vi "NI PXI-4110 Programmable Power Supply RT Driver VI.vi"(6 "Device Clock":string, 9 "Device Inputs FIFO":refnum<k33>, 11 "Device Reference":T1 format="%.0x") -> ()   [LabVIEW 2018, in "NI PXI-4110 Programmable Power Supply Custom Device.lvlib"]
uses:
  NI PXI-4110 Programmable Power Supply Custom Device.lvlib
  <vilib>/NI Veristand/Custom Device API/Custom Device Item Ref.ctl
  <vilib>/NI Veristand/Custom Device API/Custom Device Channel Type.ctl
  <vilib>/Platform/TimedLoop/XDataNode/timing_clust.ctl
  <vilib>/Platform/TimedLoop/XDataNode/nitl_modes.ctl
  <vilib>/Platform/TimedLoop/XDataNode/wakeup.ctl
  4110_Channel #.ctl
  4110_Global.vi
  <vilib>/NI Veristand/Custom Device API/Get Item Property (Boolean).vi
  <vilib>/Platform/TimedLoop/XDataNode/XDataNode.xnode
  <vilib>/Platform/TimedLoop/XDataNode/XDNodeRunTimeDep.lvlib
  <vilib>/NI VeriStand/Custom Device API/Custom Device API.lvlib
  <vilib>/NI Veristand/Custom Device Tools/Custom Device Utility Library/Custom Device Utility Library.lvlib
panel:
  in  "Status Notifier":refnum<notifier>
  # "Custom Device Template\nv1.0"
  # "Use this template as a starting point for creating a custom device code module. The input controls shown here are specially named controls that the system will use to provide the device loop with data. The controls are not required for the device loop to run. For instance, if the device doesn't produce any output data, then you don't need the Device Outputs FIFO control. If you do use these controls, however, they need to have these exact names to be functional."
  # "The optional status notifier element is used to notify the RT engine of the last state of the custom device, and to indicate the device has completed execution. If this control is not used, a default No Error value is returned to the system when the device finishes execution.\n\nNote: This error state is not checked until the system shuts down. Use an output status channel to send more immediate status values to the system."
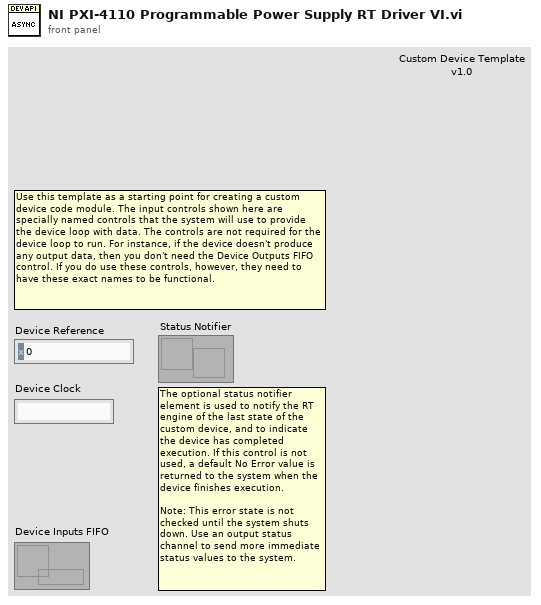
[diagram p1: front panel]
types:
  T1 = typedef "Custom Device API.lvlib/Custom Device Item Ref.ctl" = u64
  T2 = typedef "Custom Device API.lvlib/Custom Device Channel Type.ctl" = enum16{"Input", "Output"}
  T3 = typedef "Custom Device API.lvlib/Custom Device Timed Loop Priority.ctl" = enum32{"Low", "Medium", "High"}
  T4 = cluster{"instrument handle out":refnum<k15>, "Value":string, "Value":u16}[]
  T5 = typedef "XDNodeRunTimeDep.lvlib/timing_clust.ctl" = cluster{"Expected End [f-1]":u64, "Actual End [f-1]":u64, "Finished Late? [f-1]":bool, "Expected End [i-1]":u64, "Actual End [i-1]":u64, "Finished Late? [i-1]":bool, "Expected Start [i]":u64, "Actual Start [i]":u64, "Expected Start [f]":u64, "Actual Start [f]":u64, "Source Name":string, "Structure Name":string, "Period":i64, "Deadline":i64, "Offset":i64, "Start":i64, "Priority":i32, "Timeout":i32, "Mode":T6, "Wakeup Reason":T7, "Error":errorcluster, "Source Type":string, "Secondary Source Type":string, "Global End Time":u64, "Global Start Time":u64, "Frame Duration":u64, "Iteration Duration":u64, "Assigned CPU":i32, "I/O Scan Engine Mode":u32}
  T6 = typedef "XDNodeRunTimeDep.lvlib/nitl_modes.ctl" = enum32{"No Change", "Process missed periods, maintain original phase", "Discard missed periods, maintain original phase", "Process missed periods, ignore original phase", "Discard missed periods, ignore original phase"}
  T7 = typedef "XDNodeRunTimeDep.lvlib/wakeup.ctl" = enum32{"Normal", "Aborted", "Asynchronous wakeup", "Timing source error", "Timed loop error", "Timeout"}
  T8 = typedef "NI PXI-4110 Programmable Power Supply Custom Device.lvlib/4110_Channel #.ctl" = enum16{"0", "1", "2"}
  T9 = cluster{"V_min":dbl, "V_max":dbl, "I_min":dbl, "I_max":dbl}
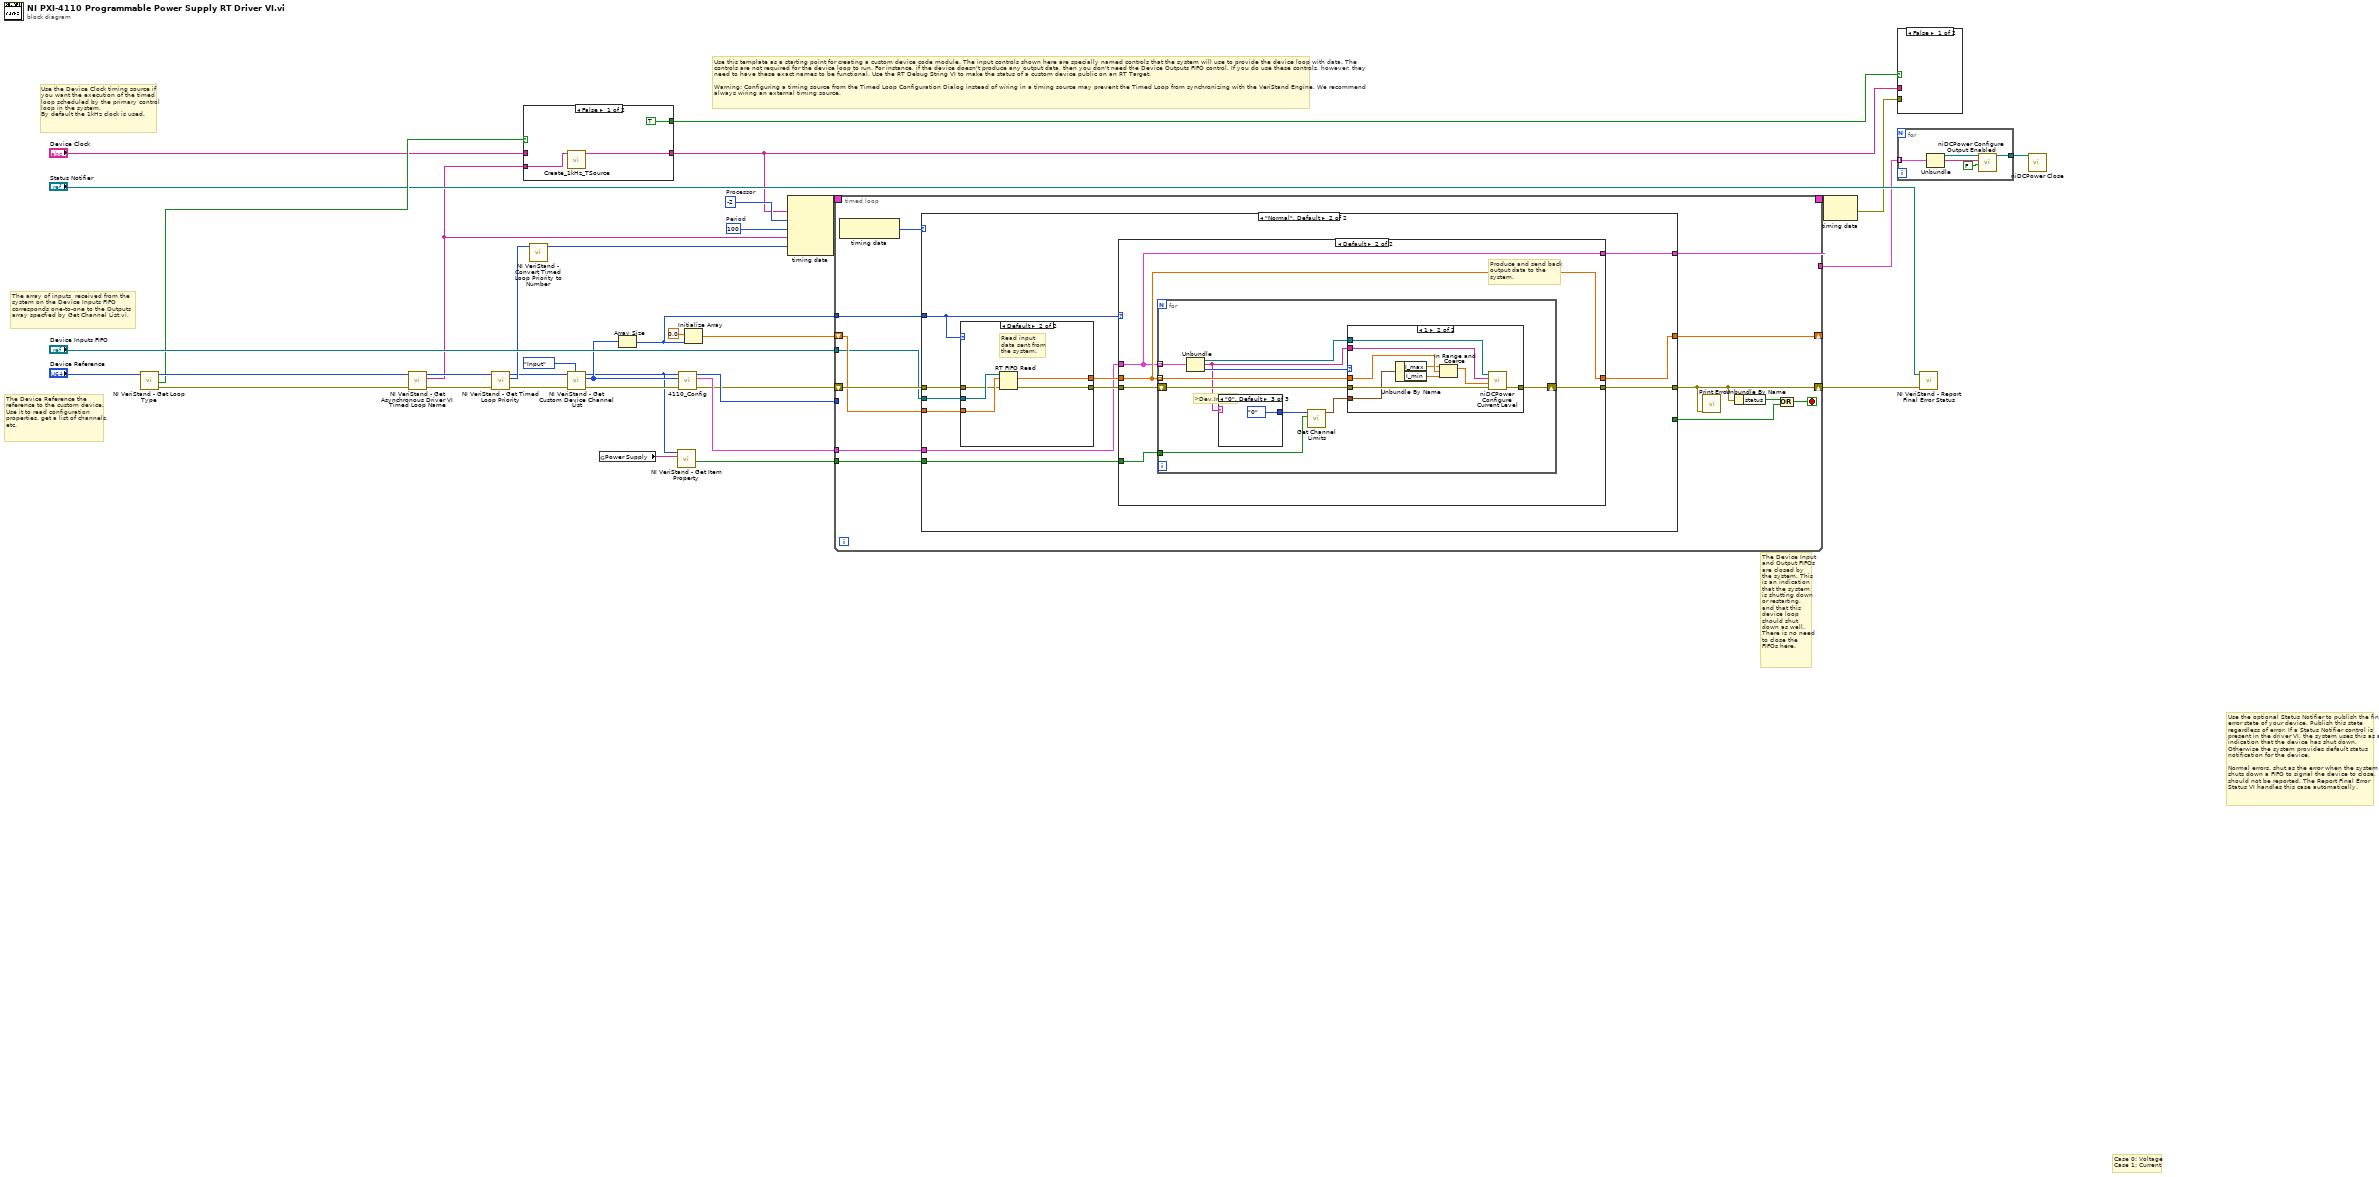
[diagram p0: block diagram]
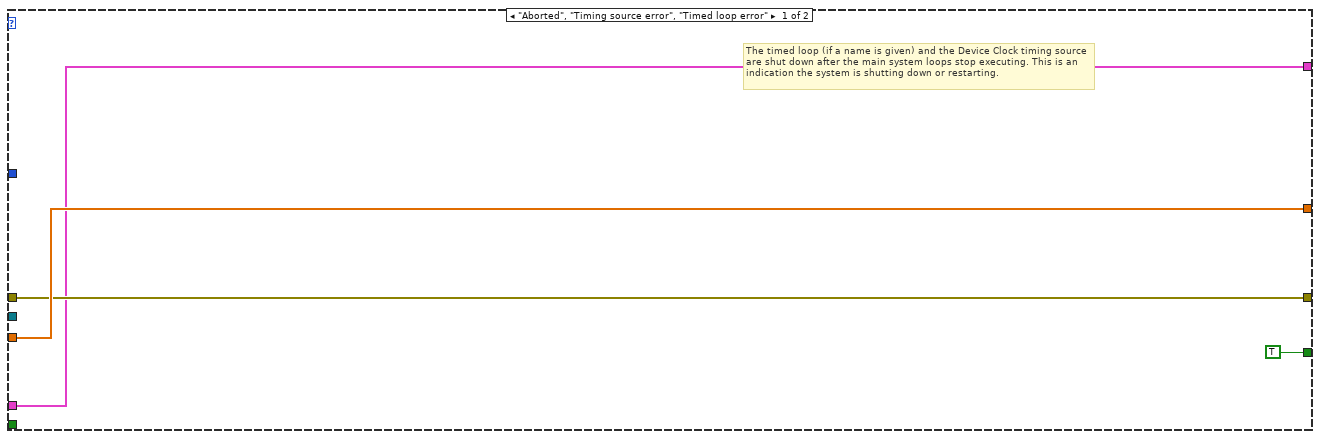
[diagram p2: hidden frame]
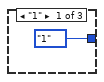
[diagram p4: hidden frame]
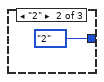
[diagram p5: hidden frame]
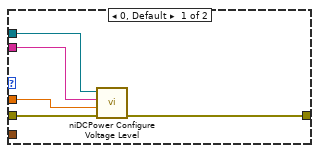
[diagram p6: hidden frame]
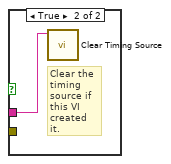
[diagram p9: hidden frame]
diagram:
  w26 = i64 100  # Period
  w27 = -2  # Processor
  # "Case 0: Voltage\nCase 1: Current"
  # "The array of inputs  received from the system on the Device Inputs FIFO corresponds one-to-one to the Outputs array specfied by Get Channel List.vi."
  # "Use the optional Status Notifier to publish the final error state of your device. Publish this state regardless of error. If a Status Notifier control is present in the driver VI, the system uses this as an indication that the device has shut down. Otherwise the system provides default status notification for the device.\n\nNormal errors, shut as the error when the system shuts down a FIFO to signal the device to close, should not be reported. The Report Final Error Status VI handles this case automatically."
  # "The Device Input and Output FIFOs are closed by the system. This is an indication that the system is shutting down or restarting, and that this device loop should shut down as well. There is no need to close the FIFOs here."
  # "The Device Reference the reference to the custom device. Use it to read configuration properties, get a list of channels, etc."
  # "Use the Device Clock timing source if you want the execution of the timed loop scheduled by the primary control loop in the system. \nBy default the 1kHz clock is used."
  # "Use this template as a starting point for creating a custom device code module. The input controls shown here are specially named controls that the system will use to provide the device loop with data. The controls are not required for the device loop to run. For instance, if the device doesn't produce any output data, then you don't need the Device Outputs FIFO control. If you do use these controls, however, they need to have these exact names to be functional. Use the RT Debug String VI to make the status of a custom device public on an RT Target.\n\nWarning: Configuring a timing source from the Timed Loop Configuration Dialog instead of wiring in a timing source may prevent the Timed Loop from synchronizing with the VeriStand Engine. We recommend always wiring an external timing source."
  n1 = call <vilib>:"NI VeriStand - Get Loop Type.vi"("Device Ref in"="Device Reference") -> ("error out"=w25:errorcluster, "Use Device Clock"=w22:bool, "Device Ref out"=w24:T1)  [unwired: 1 in, 7 out]
  n2 = call <vilib>:"NI VeriStand - Get Asynchronous Driver VI Timed Loop Name.vi"("error in (no error)"=w25, "Device Ref in"=w24) -> ("error out"=w30:errorcluster, "Device Timed Loop Name"=w16:string, "Device Ref out"=w36:T1)  [unwired: 7 out]
  n3 = call <vilib>:"NI VeriStand - Get Timed Loop Priority.vi"("error in (no error)"=w30, "Device Ref in"=w36) -> ("error out"=w4:errorcluster, "Priority"=w29:T3, "Device Ref out"=w15:T1)  [unwired: 7 out]
  n4 = case shown="False" w22 {
    tunnel: "Device Clock" -> [_ w40]
    tunnel: [w39 w40] -> w17
    tunnel: [TRUE _] -> w18
    tunnel: w16 -> [w37 _]
    frame False {
      n5 = call <vilib>:"Create_1kHz_TSource.vi"("name (in)"=w37) -> ("name (out)"=w39:string)  [unwired: 1 in, 9 out]
    }
    frame True {
    }
  }
  n6 = call <vilib>:"NI VeriStand - Convert Timed Loop Priority to Number.vi"("Priority"=w29) -> ("Numeric Priority"=w28:i32)  [unwired: 10 out]
  n7 = call <vilib>:"NI VeriStand - Get Custom Device Channel List.vi"("Channel Type"=Custom_Device_Channel_Type."Input", "error in (no error)"=w4, "Device Ref in"=w15) -> ("error out"=w12:errorcluster, "Specified Channel Ref List"=w13:T1[], "Device Ref out"=w2:T1)  [unwired: 6 out]
  n8 = global read "4110_Global.vi" "Power Supply"() -> (w3:string)
  n9 = Array Size(array=w13) -> (size(s)=w6:i32)
  n10 = call-poly <vilib>:"NI VeriStand - Get Item Property.vi"("Property Name"=w3, "Item Ref in"=w2) -> ("Value"=w1:bool)  [unwired: 6 in, 3 out]
  n11 = call "4110_Config.vi"("error in (no error)"=w12, "Specified Channel Ref List"=w13, "Device Ref out"=w2) -> ("error out"=w5:errorcluster, "Channel Info"=w11:T4, "Channel Ref List (out)"=w14:T1[])  [unwired: 6 in]
  n12 = Initialize Array(0.0 ("element"), w6) -> (w31:dbl[])
  n13 = node-c288(w17, w27, w26, w16, w28) -> (w34:T5)
  n14 = timed-loop {
    timing: w34 -> [_]
    timing-out: [_] -> w33
    shift-right: [w51] -> _
    shift-left: w31 -> [w52]
    shift-right: [w42] -> w9
    shift-left: w5 -> [w53]
    tunnel: "Device Inputs FIFO" -> [w49]
    tunnel: w6 -> [w45]
    tunnel: w14 -> [_]
    tunnel: w11 -> [w44]
    tunnel: [w43] -> w10
    tunnel: w1 -> [w41]
    stop <- w46 stop-if-true
    # ">Dev.Inputs>"
    n15 = node-c288() -> (w50:T7)  [unwired: 1 out]
    n16 = case shown="\"Normal\", Default" w50 {
      tunnel: w53 -> [w58 w65]
      tunnel: w52 -> [w59 w69]
      tunnel: [w58 w66] -> w42
      tunnel: [w59 w64] -> w51
      tunnel: w49 -> [_ w70]
      tunnel: [TRUE _] -> w47
      tunnel: w45 -> [_ w63]
      tunnel: w44 -> [w56 w62]
      tunnel: [w56 w61] -> w43
      tunnel: w41 -> [_ w60]
      frame "Aborted", "Timing source error", "Timed loop error" {
        # "The timed loop (if a name is given) and the Device Clock timing source are shut down after the main system loops stop executing. This is an indication the system is shutting down or restarting."
      }
      frame "Normal", Default {
        n17 = case shown="Default" w63 {
          tunnel: w70 -> [_ w112]
          tunnel: w69 -> [w107 w111]
          tunnel: [w107 w110] -> w68
          tunnel: [w106 w109] -> w67
          tunnel: w65 -> [w106 w108]
          frame 0 {
            # "No inputs to read\nfrom system. Inputs FIFO not created in this case, so don't write to it."
          }
          frame Default {
            # "Read input data sent from the system."
            n18 = RT FIFO Read(0:w112, 1:w111, 3:w108) -> (9:w110:dbl[], 11:w109:errorcluster)  [unwired: 4 out]
          }
        }
        n19 = case shown="Default" w63 {
          tunnel: w68 -> [w73 w78]
          tunnel: w67 -> [w72 w77]
          tunnel: [w72 w76] -> w66
          tunnel: [w73 w78] -> w64
          tunnel: w62 -> [w71 w75]
          tunnel: [w71 w75] -> w61
          tunnel: w60 -> [_ w74]
          frame 0 {
            # "No outputs to write to system. The Device Outputs FIFO is never created in this case, so don't write to it."
          }
          frame Default {
            # "Produce and send back output data to the system."
            n20 = for {
              tunnel: w75 -> [w88] mode=indexing
              tunnel: w78 -> [w83] mode=indexing
              shift-right: [w85] -> w76
              shift-left: w77 -> [w86]
              tunnel: w74 -> [w79]
              n21 = Unbundle(w88) -> ("instrument handle out"=w87:refnum<k15>, "Value"=w82:string, "Value"=w84:u16)
              n22 = case shown="\"0\", Default" w82 {
                tunnel: [4110_Channel_#."1" ("Channel #") 4110_Channel_#."2" ("Channel #") 4110_Channel_#."0" ("Channel #")] -> w81
                frame "1" {
                }
                frame "2" {
                }
                frame "0", Default {
                }
              }
              n23 = call "Get Channel Limits.vi"("External Supply?"=w79, "Channel #"=w81) -> ("output cluster"=w80:T9)  [unwired: 8 in, 1 out]
              n24 = case shown="1" w84 {
                tunnel: w87 -> [w96 w105]
                tunnel: w82 -> [w93 w103]
                tunnel: w83 -> [w95 w102]
                tunnel: w86 -> [w94 w104]
                tunnel: [w92 w97] -> w85
                tunnel: w80 -> [_ w100]
                frame 0, Default {
                  n25 = call <instrlib>:"niDCPower Configure Voltage Level.vi"("error in (no error)"=w94, "voltage level"=w95, "channel name"=w93, "instrument handle"=w96) -> ("error out"=w92:errorcluster)  [unwired: 6 in, 1 out]
                }
                frame 1 {
                  n26 = Unbundle By Name(w100) -> ("I_max"=w99:dbl, "I_min"=w98:dbl)
                  n27 = In Range and Coerce(upper limit=w99, x=w102, lower limit=w98) -> (coerced(x)=w101:dbl)  [unwired: 1 out]
                  n28 = call <instrlib>:"niDCPower Configure Current Level.vi"("error in (no error)"=w104, "current level"=w101, "channel name"=w103, "instrument handle"=w105) -> ("error out"=w97:errorcluster)  [unwired: 6 in, 1 out]
                }
              }
            }
          }
        }
      }
    }
    n29 = call "Print Error.vi"("error out"=w42) -> ()  [unwired: 10 in]
    n30 = Unbundle By Name(w42) -> ("status"=w48:bool)
    n31 = Compound Arithmetic op=OR(w48, w47) -> (w46:bool)
  }
  n32 = node-c288(w33) -> (w19:errorcluster)
  n33 = case shown="False" w18 {
    tunnel: w19 -> [_ _]
    tunnel: w17 -> [_ w114]
    frame False {
    }
    frame True {
      # "Clear the timing source if this VI created it."
      n34 = call <vilib>:"Clear Timing Source.vi"("name"=w114) -> ()  [unwired: 1 in, 10 out]
    }
  }
  n35 = for {
    tunnel: w10 -> [w119] mode=indexing
    tunnel: [w115] -> w7
    n36 = Unbundle(w119) -> ("instrument handle out"=w118:refnum<k15>, "Value"=w117:string)  [unwired: 1 out]
    n37 = call <instrlib>:"niDCPower Configure Output Enabled.vi"("output enabled"=FALSE, "channel name"=w117, "instrument handle"=w118) -> ("instrument handle out"=w115:refnum<k15>)  [unwired: 7 in, 1 out]
  }
  n38 = call <vilib>:"NI VeriStand - Report Final Error Status.vi"("error in (no error)"=w9, "Status Notifier"="Status Notifier") -> ()  [unwired: 1 in, 9 out]
  n39 = call <instrlib>:"niDCPower Close.vi"("instrument handle"=w7) -> ()  [unwired: 10 in, 1 out]
